vi "RSZVB Get IMOD Measurement Order.vi"(8 "error in (no error)":errorcluster {"code" format="%.0x"}, 9 "Product Order (3)":i32(ring)=3 items=["3"=3, "5"=5, "7"=7, "9"=9], 10 "Channel (1)":i32=1, 11 "VISA session":refnum<visa-resource-name>) -> (0 "error out":errorcluster {"code" format="%.0x"}, 1 "Measurement State":bool, 3 "dup VISA session":refnum<visa-resource-name>)   [LabVIEW 2011]
doc: "This VI returns the state of the measurement of the intermodulation products of order <IM order>.\n\nNote(s):\n\n(1) This VI is not available for R&S ZVB instrument.\n\nRemote-control command(s):\n[SENSe<Ch>:]FREQuency:IMODulation:ORDer<Im>[:STATe]?"
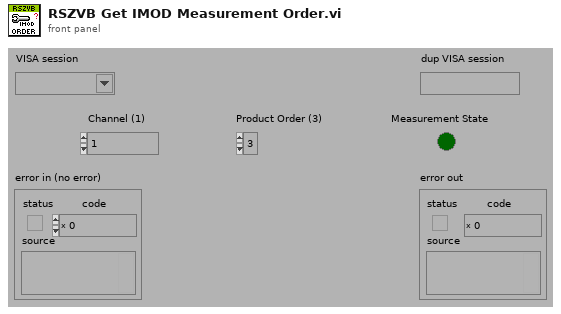
[diagram p1: front panel]
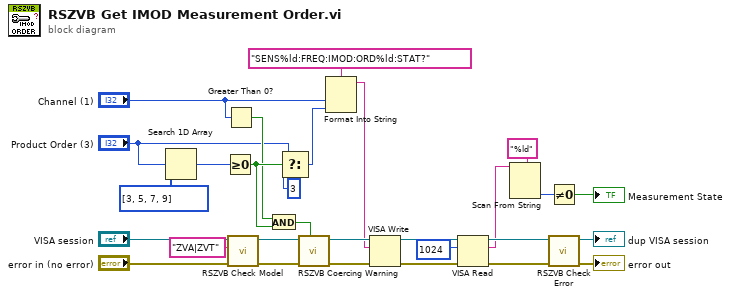
[diagram p0: block diagram]
diagram:
  n1 = Search 1D Array(1D array=i32[] [3, 5, 7, 9], element="Product Order (3)") -> (index of element=w29:i32)  [unwired: 1 in]
  n2 = Greater Or Equal To 0?(x=w29) -> (x >= 0?=w26:bool)
  n3 = Greater Than 0?(x="Channel (1)") -> (x > 0?=w24:bool)
  n4 = call "RSZVB Check Model.vi"("error in (no error)"="error in (no error)", "Model"="ZVA|ZVT", "VISA session"="VISA session") -> ("error out"=w1:errorcluster, "dup VISA session"=w2:refnum<visa-resource-name>)  [unwired: 7 in]
  n5 = And(x=w24, y=w26) -> (x .and. y?=w25:bool)
  n6 = Select(t="Product Order (3)", s=w26, f=3) -> (s? t:f=w28:i32)
  n7 = call "RSZVB Coercing Warning.vi"("In Range?"=w25, "error in (no error)"=w1, "VISA session"=w2) -> ("error out"=w20:errorcluster, "dup VISA session"=w21:refnum<visa-resource-name>)  [unwired: 7 in]
  n8 = Format Into String(format string="SENS%ld:FREQ:IMOD:ORD%ld:STAT?", "Channel (1)", w28) -> (resulting string=w19:string)  [unwired: 2 in, 1 out]
  n9 = VISA Write(VISA resource name=w21, write buffer=w19, error in (no error)=w20) -> (VISA resource name out=w14:refnum<visa-resource-name>, error out=w13:errorcluster)  [unwired: 1 out]
  n10 = VISA Read(VISA resource name=w14, byte count=u32 1024 ("byte count (0)"), error in (no error)=w13) -> (VISA resource name out=w11:refnum<visa-resource-name>, read buffer=w6:string, error out=w10:errorcluster)  [unwired: 1 out]
  n11 = Scan From String(format string="%ld", input string=w6) -> (output 1=w8:i32)  [unwired: 3 in, 3 out]
  n12 = Not Equal To 0?(x=w8) -> (x != 0?=→"Measurement State":bool)
  n13 = call "RSZVB Check Error.vi"("error in (no error)"=w10, "VISA session"=w11) -> ("error out"=→"error out":errorcluster, "dup VISA session"=→"dup VISA session":refnum<visa-resource-name>)  [unwired: 8 in]
